vi "Example_SignalEntity.vi"() -> ()   [LabVIEW 2021, in "BrainStem2_LabVIEW_Library.lvlib"]
uses:
  BrainStem2_LabVIEW_Library.lvlib
panel:
  out "Get Output:\nT2 Time (nano-seconds)":u32
  out "Get Output:\nT3 Time (nano-seconds)":u32
  out "Get Input:\nCalculated Duty Cycle":dbl
  out "Get Input:\nT2 Time (nano-seconds)":u32
  out "Get Input:\nT3 Time (nano-seconds)":u32
  in  "Set Output:\nT2 Time (nano-seconds)":u32=50000000
  in  "Set Output:\nT3 Time (nano-seconds)":u32=100000000
  # "Signal Entity Example for the MTMUSBStem"
  # "Signal Output - Digital Enity/Pin 6 - Signal Entity 2"
  # "Signal Input - Digital Enity/Pin 4 - Signal Entity 0"
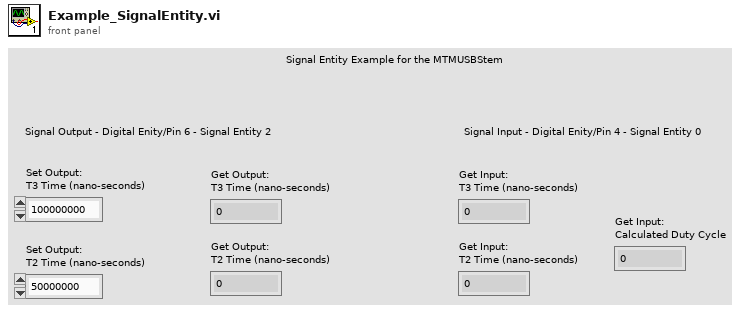
[diagram p1: front panel]
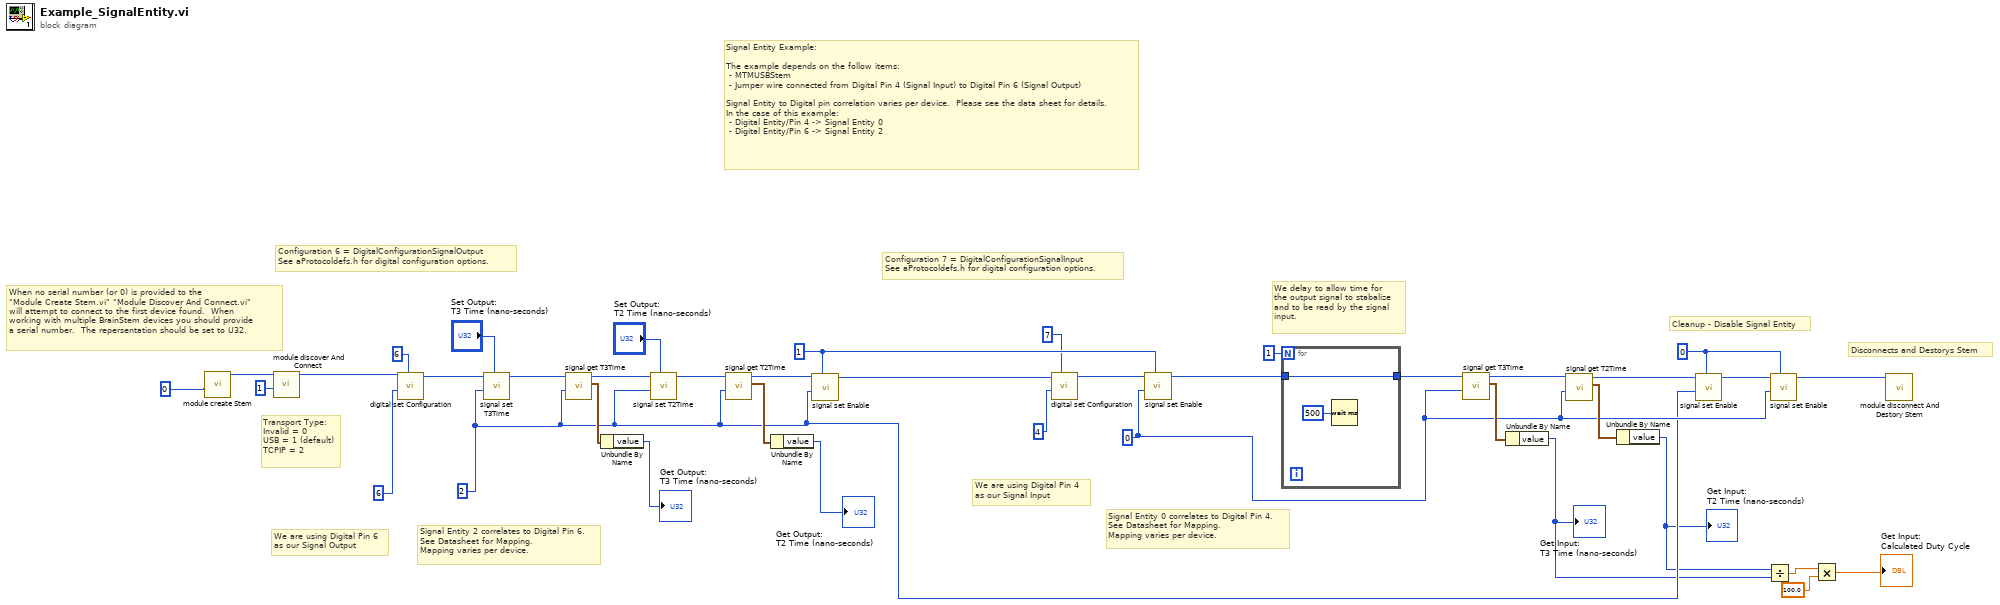
[diagram p0: block diagram]
diagram:
  w15 = 0 ("enable")
  w8 = 0 ("signalNum")
  w24 = 1 ("enable")
  w7 = 2 ("signalNum")
  # "Signal Entity Example:\n\nThe example depends on the follow items:\n - MTMUSBStem\n - Jumper wire connected from Digital Pin 4 (Signal Input) to Digital Pin 6 (Signal Output)\n\nSignal Entity to Digital pin correlation varies per device.  Please see the data sheet for details.\nIn the case of this example: \n - Digital Entity/Pin 4 -> Signal Entity 0\n - Digital Entity/Pin 6 -> Signal Entity 2"
  # "Cleanup - Disable Signal Entity"
  # "Disconnects and Destorys Stem"
  # "Signal Entity 0 correlates to Digital Pin 4.\nSee Datasheet for Mapping.\nMapping varies per device."
  # "We are using Digital Pin 4\nas our Signal Input"
  # "Configuration 7 = DigitalConfigurationSignalInput\nSee aProtocoldefs.h for digital configuration options."
  # "We delay to allow time for\nthe output signal to stabalize\nand to be read by the signal \ninput."
  # "Configuration 6 = DigitalConfigurationSignalOutput\nSee aProtocoldefs.h for digital configuration options."
  # "We are using Digital Pin 6\nas our Signal Output"
  # "Signal Entity 2 correlates to Digital Pin 6.\nSee Datasheet for Mapping.\nMapping varies per device."
  # "When no serial number (or 0) is provided to the\n\"Module Create Stem.vi\" \"Module Discover And Connect.vi\"\nwill attempt to connect to the first device found.  When \nworking with multiple BrainStem devices you should provide\na serial number.  The repersentation should be set to U32."
  # "Transport Type:\nInvalid = 0\nUSB = 1 (default)\nTCPIP = 2"
  n1 = call "module create Stem.vi"("sn"=u32 0) -> ("id out"=w39:u32)  [unwired: 8 in, 2 out]
  n2 = call "module discover And Connect.vi"("transport"=1, "id"=w39) -> ("id out"=w28:u32)  [unwired: 7 in, 2 out]
  n3 = call "digital set Configuration.vi"("configuration"=6, "index"=6 ("digitalNum"), "id"=w28) -> ("id out"=w27:u32)  [unwired: 6 in, 2 out]
  n4 = call "signal set T3Time.vi"("t3_nsec"="Set Output:\nT3 Time (nano-seconds)", "index"=w7, "id"=w27) -> ("id out"=w37:u32)  [unwired: 6 in, 2 out]
  n5 = call "signal get T3Time.vi"("index"=w7, "id"=w37) -> ("result out"=w32:cluster{"value":i32, "error":i32}, "id out"=w36:u32)  [unwired: 7 in, 1 out]
  n6 = Unbundle By Name(w32) -> ("value"=→"Get Output:\nT3 Time (nano-seconds)":i32)
  n7 = call "signal set T2Time.vi"("t2_nsec"="Set Output:\nT2 Time (nano-seconds)", "index"=w7, "id"=w36) -> ("id out"=w35:u32)  [unwired: 6 in, 2 out]
  n8 = call "signal get T2Time.vi"("index"=w7, "id"=w35) -> ("result out"=w31:cluster{"value":i32, "error":i32}, "id out"=w26:u32)  [unwired: 7 in, 1 out]
  n9 = Unbundle By Name(w31) -> ("value"=→"Get Output:\nT2 Time (nano-seconds)":i32)
  n10 = call "signal set Enable.vi"("enable"=w24, "index"=w7, "id"=w26) -> ("id out"=w4:u32)  [unwired: 6 in, 2 out]
  n11 = call "digital set Configuration.vi"("configuration"=7, "index"=4 ("digitalNum"), "id"=w4) -> ("id out"=w23:u32)  [unwired: 6 in, 2 out]
  n12 = call "signal set Enable.vi"("enable"=w24, "index"=w8, "id"=w23) -> ("id out"=w19:u32)  [unwired: 6 in, 2 out]
  n13 = for {
    N: 1 -> [_]
    tunnel: [w40] -> w20
    tunnel: w19 -> [w40]
    n14 = Wait (ms)(milliseconds to wait=u32 500) -> ()  [unwired: 1 out]
  }
  n15 = call "signal get T3Time.vi"("index"=w8, "id"=w20) -> ("result out"=w18:cluster{"value":i32, "error":i32}, "id out"=w16:u32)  [unwired: 7 in, 1 out]
  n16 = Unbundle By Name(w18) -> ("value"=w3:i32)
  "Get Input:\nT3 Time (nano-seconds)" <- w3
  n17 = call "signal get T2Time.vi"("index"=w8, "id"=w16) -> ("result out"=w17:cluster{"value":i32, "error":i32}, "id out"=w14:u32)  [unwired: 7 in, 1 out]
  n18 = Unbundle By Name(w17) -> ("value"=w2:i32)
  "Get Input:\nT2 Time (nano-seconds)" <- w2
  n19 = call "signal set Enable.vi"("enable"=w15, "index"=w7, "id"=w14) -> ("id out"=w13:u32)  [unwired: 6 in, 2 out]
  n20 = Divide(x=w2, y=w3) -> (x/y=w11:dbl)
  n21 = call "signal set Enable.vi"("enable"=w15, "index"=w8, "id"=w13) -> ("id out"=w12:u32)  [unwired: 6 in, 2 out]
  n22 = Multiply(x=w11, y=100.0) -> (x*y=→"Get Input:\nCalculated Duty Cycle":dbl)
  n23 = call "module disconnect And Destory Stem.vi"("id"=w12) -> ()  [unwired: 8 in, 3 out]
